vi "GlobalExitVar.vi"() -> ()   [LabVIEW 2013]
panel:
  in  "Emergency Exit":bool
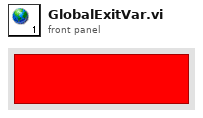
[diagram p1: front panel]
diagram:
